vi "Generate_PWM.vi"(1 "Balance_PWM":dbl, 2 "Position_PWM":dbl) -> (0 "PWM":dbl)   [LabVIEW 2018]
uses:
  Global_variables.vi
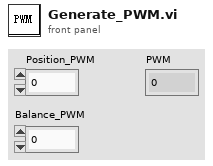
[diagram p1: front panel]
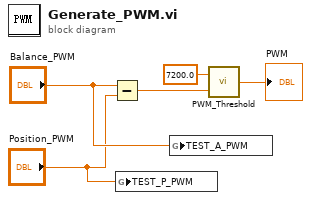
[diagram p0: block diagram]
diagram:
  n1 = Subtract(x="Balance_PWM", y="Position_PWM") -> (x-y=w5:dbl)
  n2 = global write "Global_variables.vi" "TEST_P_PWM"("Position_PWM") -> ()
  n3 = global write "Global_variables.vi" "TEST_A_PWM"("Balance_PWM") -> ()
  n4 = call "PWM_Threshold.vi"("Input_PWM"=w5, "Threshold"=7200.0) -> ("Trimmed_PWM"=→"PWM":dbl)
